vi "Benchmark FP local.vi"() -> ()   [LabVIEW 2016]
panel:
  out "x+y":i32
  out "us/iteration":dbl format="%.6f"
  in  "iterations":i32=1000000000
  # "0.053144 us/iteration 1E9 iterations"
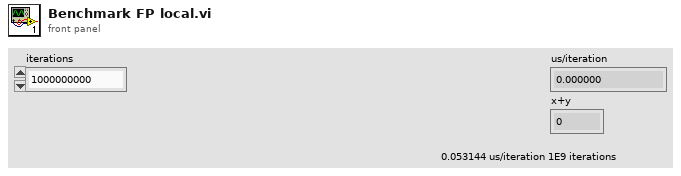
[diagram p1: front panel]
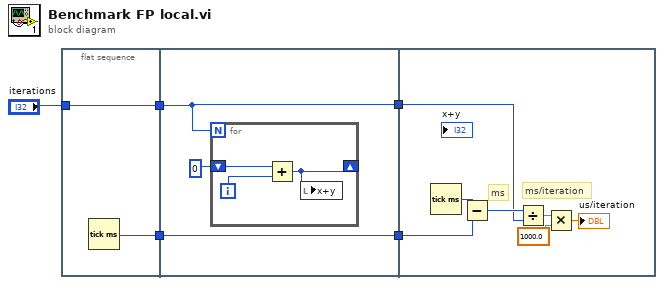
[diagram p0: block diagram]
diagram:
  n1 = flat-sequence {
    tunnel: [w7] -> w5
    tunnel: [w6] -> w2
    tunnel: "iterations" -> [w6]
    tunnel: w5 -> [w10]
    tunnel: [w10] -> w4
    tunnel: [w9] -> w3
    tunnel: w2 -> [w9]
    tunnel: w4 -> [w19]
    tunnel: w3 -> [w17]
    frame #0 {
      n2 = Tick Count (ms)() -> (millisecond timer value=w7:u32)
    }
    frame #1 {
      n3 = for {
        N: w9 -> [_]
        shift-right: [w11] -> _
        shift-left: 0 -> [w12]
        i -> [w13]
        n4 = Add(x=w12, y=w13) -> (x+y=w11:i32)
        n5 = local write "x+y"(w11) -> ()
      }
    }
    frame #2 {
      # "ms/iteration"
      # "ms"
      n6 = Tick Count (ms)() -> (millisecond timer value=w20:u32)
      n7 = Subtract(x=w20, y=w19) -> (x-y=w18:u32)
      n8 = Divide(x=w18, y=w17) -> (x/y=w16:dbl)
      n9 = Multiply(x=w16, y=1000.0) -> (x*y=→"us/iteration":dbl)
    }
  }
